vi "GetParameters.vi"() -> ()   [LabVIEW 2019]
panel:
  in  "Particle Measurements () ( Analysis 1) 2":dbl[][](array[numeric])=[[-56.76927788622368, -45.1835918273996, 105.49419358199933], [-30.750625061451895, -44.325520815009625, 68.38552020511543], [-2.1334363725101984, -41.244912471531386, 76.37528039980916], [29.421996518985512, -37.122571270909646, 66.76480625926112], [60.274191851517, -32.079988846679804, 77.89870639104257], [-27.384001212853015, -15.978175056162065, 86.41531854069336], [-57.12939186077779, -13.03821655068185, 95.19110987959867], [0.8157806454249426, -11.537585106806365, 62.65946754704529], [64.98159237148258, -10.313960473940636, 69.99468128482164], [32.817069309857175, -8.540823667699138, 60.761895469821624], [-27.702412887676708, 9.579157204985355, 75.19141634191074], [37.70198789537908, 10.266392184363795, 79.57588918149607], [4.765820750936916, 14.081942717017705, 68.51007357972752], [70.76309958374665, 15.0790537252041, 75.75366895030213], [-57.414383042714164, 15.41503234985349, 118.75231783795783], [38.63309694823678, 26.53758397944904, 71.30269833859165], [6.772199998928159, 31.011934793632058, 85.69802266359905], [73.41514437007658, 32.69142082569389, 70.93244311358723], [-24.768202720713113, 34.61278172695657, 103.9423369146022], [-57.24809342732071, 38.73521730856287, 115.82572787967626], [44.20007179514008, 45.43219064427871, 19.51567546366857], [79.96818037855478, 49.88188093239065, 32.063710672745785], [8.120161023706626, 52.661005797649594, 173.15722658736857], [-57.72569267153209, 55.966495303633685, 93.82758352841635], [-23.250568280228087, 59.94125217156932, 90.95001222194976]] format="%.2f"
  out "appended array 3":cluster{dbl, dbl}[][](array[cluster])
  out "MatrixPoint":cluster{dbl, dbl}[][](array[cluster])
  out "appended array":cluster{"X":dbl, "Y":dbl}[][](array[cluster])
  out "Number of Particles":i32
  out "CalImgOut":T1(plugin-control)
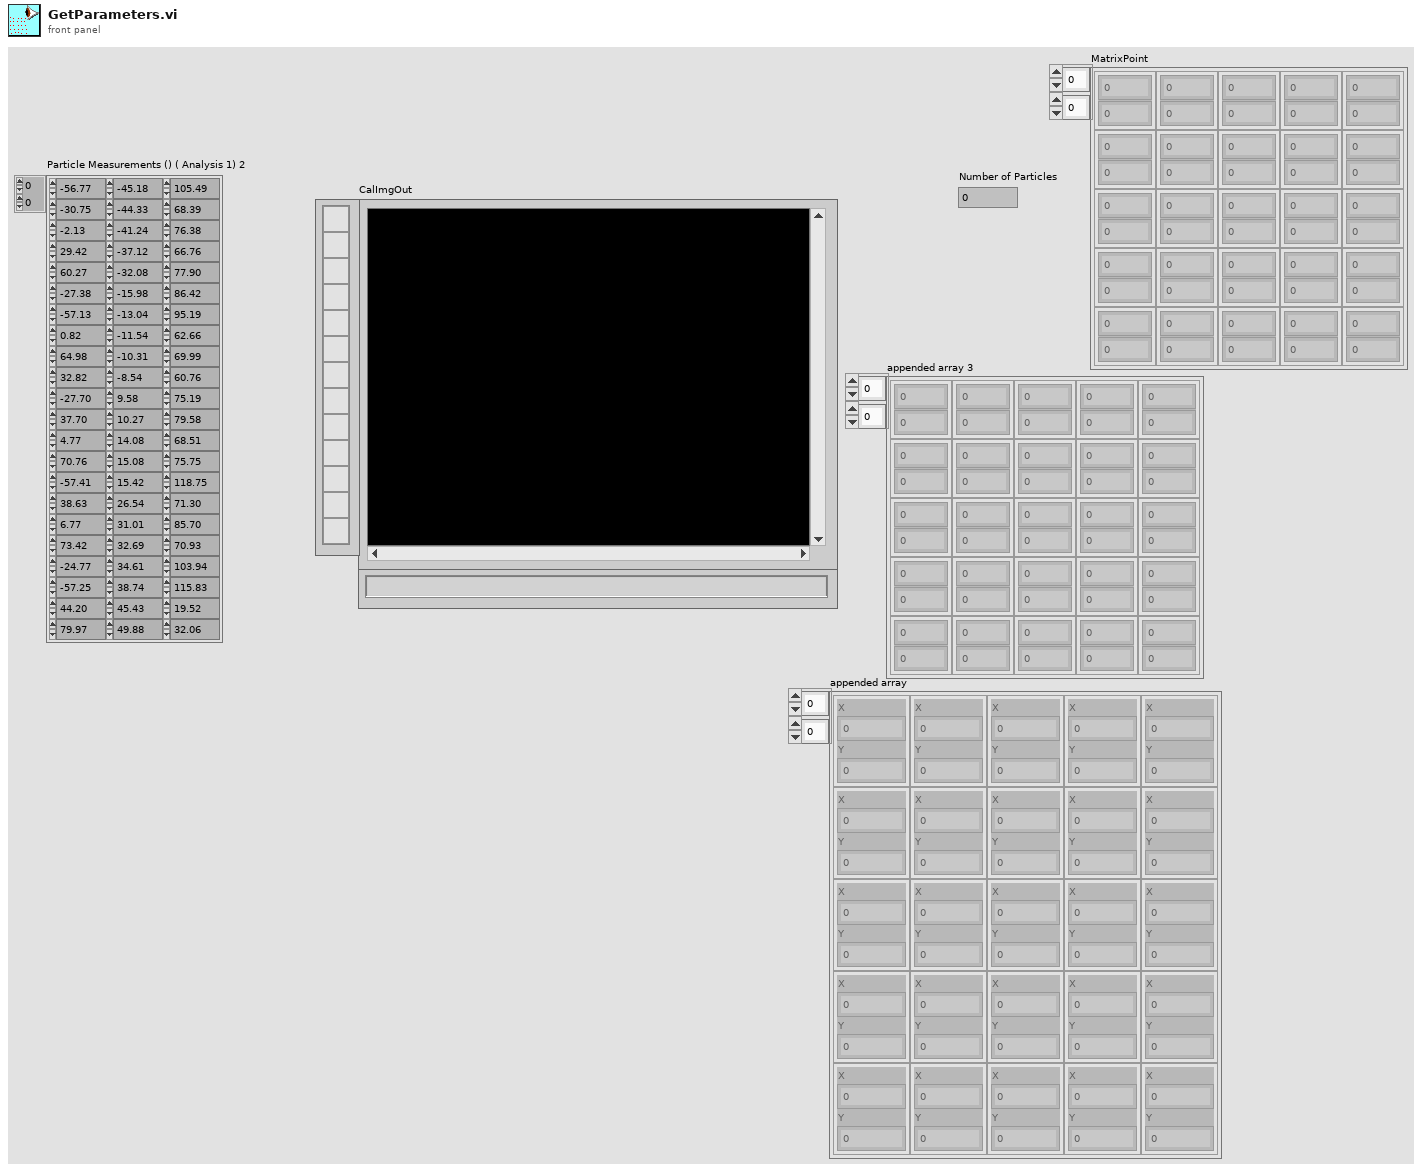
[diagram p1: front panel]
types:
  T1 = typedef "IMAQ Image.ctl" = refnum<image>
  T2 = typedef "Image Type" = u32
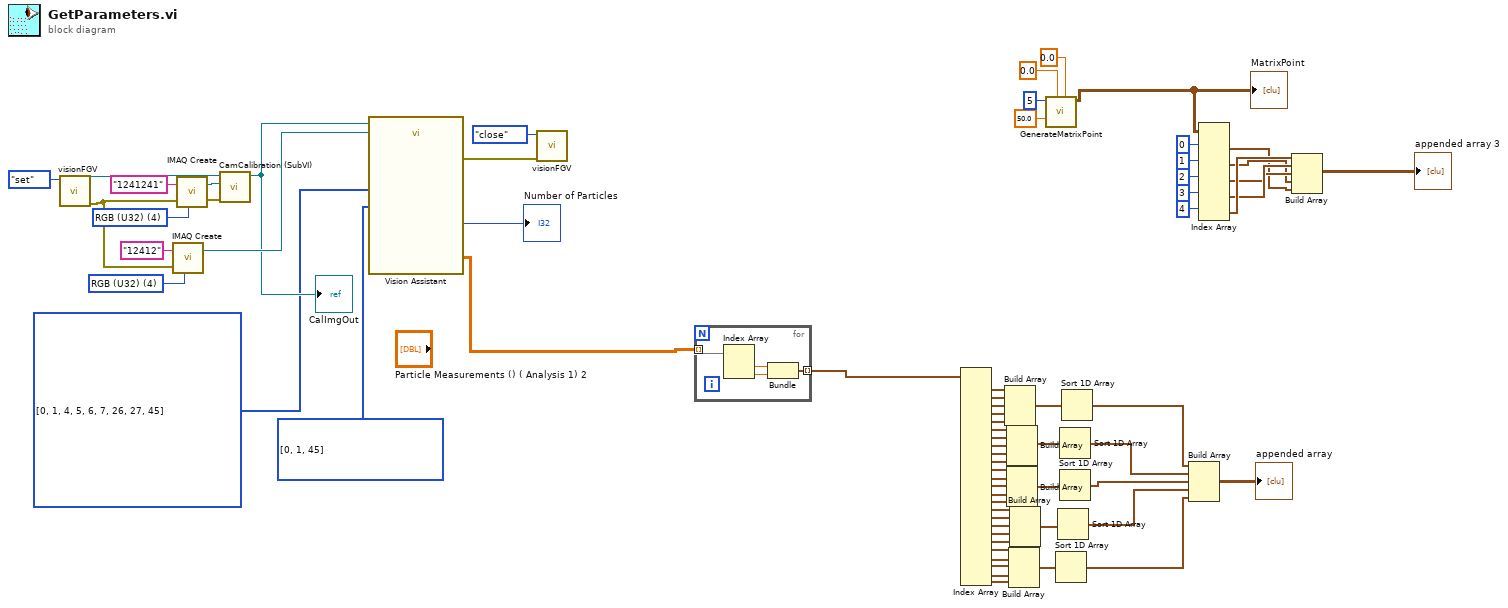
[diagram p0: block diagram]
diagram:
  w55 = i32[] [0, 1, 45] items=["Center of Mass X", "Center of Mass Y", "First Pixel X", "First Pixel Y", "Bounding Rect Left", "Bounding Rect Top", "Bounding Rect Right", "Bounding Rect Bottom", "Max Feret Diameter Start X", "Max Feret Diameter Start Y", "Max Feret Diameter End X", "Max Feret Diameter End Y", "Max Horiz. Segment Length Left", "Max Horiz. Segment Length Right", "Max Horiz. Segment Length Row", "-", "Bounding Rect Width", "Bounding Rect Height", "Bounding Rect Diagonal", "Perimeter", "Convex Hull Perimeter", "Holes' Perimeter", "Max Feret Diameter", "Equivalent Ellipse Major Axis", "Equivalent Ellipse Minor Axis", "Equivalent Ellipse Minor Axis (Feret)", "Equivalent Rect Long Side", "Equivalent Rect Short Side", "Equivalent Rect Diagonal", "Equivalent Rect Short Side (Feret)", "Average Horiz. Segment Length", "Average Vert. Segment Length", "Hydraulic Radius", "Waddel Disk Diameter", "-", "Area", "Holes' Area", "Particle & Holes' Area", "Convex Hull Area", "Image Area", "-", "Number of Holes", "Number of Horiz. Segments", "Number of Vert. Segments", "-", "Orientation", "Max Feret Diameter Orientation", "-", "% Area/Image Area", "% Area/(Particle & Holes' Area)", "Ratio of Equivalent Ellipse Axes", "Ratio of Equivalent Rect Sides", "-", "Elongation Factor", "Compactness Factor", "Heywood Circularity Factor", "Type Factor", "-", "Sum X", "Sum Y", "Sum XX", "Sum XY", "Sum YY", "Sum XXX", "Sum XXY", "Sum XYY", "Sum YYY", "-", "Moment of Inertia XX", "Moment of Inertia XY", "Moment of Inertia YY", "Moment of Inertia XXX", "Moment of Inertia XXY", "Moment of Inertia XYY", "Moment of Inertia YYY", "Norm. Moment of Inertia XX", "Norm. Moment of Inertia XY", "Norm. Moment of Inertia YY", "Norm. Moment of Inertia XXX", "Norm. Moment of Inertia XXY", "Norm. Moment of Inertia XYY", "Norm. Moment of Inertia YYY", "Hu Moment 1", "Hu Moment 2", "Hu Moment 3", "Hu Moment 4", "Hu Moment 5", "Hu Moment 6", "Hu Moment 7"] ("Real-World Measurements (Particle Analysis 1)")
  w56 = i32[] [0, 1, 4, 5, 6, 7, 26, 27, 45] items=["Center of Mass X", "Center of Mass Y", "First Pixel X", "First Pixel Y", "Bounding Rect Left", "Bounding Rect Top", "Bounding Rect Right", "Bounding Rect Bottom", "Max Feret Diameter Start X", "Max Feret Diameter Start Y", "Max Feret Diameter End X", "Max Feret Diameter End Y", "Max Horiz. Segment Length Left", "Max Horiz. Segment Length Right", "Max Horiz. Segment Length Row", "-", "Bounding Rect Width", "Bounding Rect Height", "Bounding Rect Diagonal", "Perimeter", "Convex Hull Perimeter", "Holes' Perimeter", "Max Feret Diameter", "Equivalent Ellipse Major Axis", "Equivalent Ellipse Minor Axis", "Equivalent Ellipse Minor Axis (Feret)", "Equivalent Rect Long Side", "Equivalent Rect Short Side", "Equivalent Rect Diagonal", "Equivalent Rect Short Side (Feret)", "Average Horiz. Segment Length", "Average Vert. Segment Length", "Hydraulic Radius", "Waddel Disk Diameter", "-", "Area", "Holes' Area", "Particle & Holes' Area", "Convex Hull Area", "Image Area", "-", "Number of Holes", "Number of Horiz. Segments", "Number of Vert. Segments", "-", "Orientation", "Max Feret Diameter Orientation", "-", "% Area/Image Area", "% Area/(Particle & Holes' Area)", "Ratio of Equivalent Ellipse Axes", "Ratio of Equivalent Rect Sides", "-", "Elongation Factor", "Compactness Factor", "Heywood Circularity Factor", "Type Factor", "-", "Sum X", "Sum Y", "Sum XX", "Sum XY", "Sum YY", "Sum XXX", "Sum XXY", "Sum XYY", "Sum YYY", "-", "Moment of Inertia XX", "Moment of Inertia XY", "Moment of Inertia YY", "Moment of Inertia XXX", "Moment of Inertia XXY", "Moment of Inertia XYY", "Moment of Inertia YYY", "Norm. Moment of Inertia XX", "Norm. Moment of Inertia XY", "Norm. Moment of Inertia YY", "Norm. Moment of Inertia XXX", "Norm. Moment of Inertia XXY", "Norm. Moment of Inertia XYY", "Norm. Moment of Inertia YYY", "Hu Moment 1", "Hu Moment 2", "Hu Moment 3", "Hu Moment 4", "Hu Moment 5", "Hu Moment 6", "Hu Moment 7"] ("Pixel Measurements (Particle Analysis 1)")
  w68 = T2 4 items=["Grayscale (U8)", "Grayscale (I16)", "Grayscale (SGL)", "Complex (CSG)", "RGB (U32)", "HSL (U32)", "RGB (U64)", "Grayscale (U16)"] ("Image Type")
  w69 = T2 4 items=["Grayscale (U8)", "Grayscale (I16)", "Grayscale (SGL)", "Complex (CSG)", "RGB (U32)", "HSL (U32)", "RGB (U64)", "Grayscale (U16)"] ("Image Type")
  n1 = call "visionFGV.vi"("Function"=enum16{"set", "read", "close"}."set") -> ("error out"=w63:errorcluster, "Image Out fgv"=w61:T1)  [unwired: 9 in]
  n2 = call "IMAQ Create"("Image Name"="12412", "Image Type"=w68, "error in (no error)"=w63) -> ("New Image"=w66:T1)  [unwired: 2 in, 1 out]
  n3 = call "IMAQ Create"("Image Name"="1241241", "Image Type"=w69, "error in (no error)"=w63) -> ("New Image"=w65:T1, "error out"=w62:errorcluster)  [unwired: 2 in]
  n4 = call "CamCalibration (SubVI).vi"("error in"=w62, "Image Dst"=w65, "Image In"=w61) -> ("Image Out"=w60:T1)  [unwired: 7 in, 1 out]
  "CalImgOut" <- w60
  n5 = call "Vision Assistant"("Image In"=w60, "Image Dst"=w66, "Pixel Measurements (Particle Analysis 1)"=w56, "Real-World Measurements (Particle Analysis 1)"=w55) -> ("Particle Measurements (Real-World) (Particle Analysis 1)"=w1:dbl[][], "Number of Particles (Particle Analysis 1)"=→"Number of Particles":i32, "error out"=w59:errorcluster)  [unwired: 19 in, 2 out]
  n6 = call "visionFGV.vi"("Error In"=w59, "Function"=enum16{"set", "read", "close"}."close") -> ()  [unwired: 8 in, 2 out]
  n7 = for {
    tunnel: w1 -> [w74] mode=indexing
    tunnel: [w71] -> w27 mode=indexing
    n8 = Index Array(array=w74) -> (element #1=w73:dbl, element #2=w72:dbl)  [unwired: 2 in]
    n9 = Bundle("Numeric"=w73, "Numeric"=w72) -> (w71:cluster{"Numeric":dbl, "Numeric":dbl})  [unwired: 1 in]
  }
  n10 = Index Array(array=w27) -> (element #1=w28:cluster{"Numeric":dbl, "Numeric":dbl}, element #2=w38:cluster{"Numeric":dbl, "Numeric":dbl}, element #3=w37:cluster{"Numeric":dbl, "Numeric":dbl}, element #4=w36:cluster{"Numeric":dbl, "Numeric":dbl}, element #5=w35:cluster{"Numeric":dbl, "Numeric":dbl}, element #6=w34:cluster{"Numeric":dbl, "Numeric":dbl}, element #7=w33:cluster{"Numeric":dbl, "Numeric":dbl}, element #8=w30:cluster{"Numeric":dbl, "Numeric":dbl}, element #9=w32:cluster{"Numeric":dbl, "Numeric":dbl}, element #10=w31:cluster{"Numeric":dbl, "Numeric":dbl}, element #11=w24:cluster{"Numeric":dbl, "Numeric":dbl}, element #12=w23:cluster{"Numeric":dbl, "Numeric":dbl}, element #13=w22:cluster{"Numeric":dbl, "Numeric":dbl}, element #14=w21:cluster{"Numeric":dbl, "Numeric":dbl}, element #15=w20:cluster{"Numeric":dbl, "Numeric":dbl}, element #16=w19:cluster{"Numeric":dbl, "Numeric":dbl}, element #17=w18:cluster{"Numeric":dbl, "Numeric":dbl}, element #18=w17:cluster{"Numeric":dbl, "Numeric":dbl}, element #19=w16:cluster{"Numeric":dbl, "Numeric":dbl}, element #20=w15:cluster{"Numeric":dbl, "Numeric":dbl}, element #21=w14:cluster{"Numeric":dbl, "Numeric":dbl}, element #22=w13:cluster{"Numeric":dbl, "Numeric":dbl}, element #23=w12:cluster{"Numeric":dbl, "Numeric":dbl}, element #24=w11:cluster{"Numeric":dbl, "Numeric":dbl}, element #25=w10:cluster{"Numeric":dbl, "Numeric":dbl})  [unwired: 25 in]
  n11 = Build Array(w28, w38, w37, w36, w35) -> (w26:cluster{"Numeric":dbl, "Numeric":dbl}[])
  n12 = Build Array(w34, w33, w30, w32, w31) -> (w25:cluster{"Numeric":dbl, "Numeric":dbl}[])
  n13 = Build Array(w24, w23, w22, w21, w20) -> (w7:cluster{"Numeric":dbl, "Numeric":dbl}[])
  n14 = Build Array(w14, w13, w12, w11, w10) -> (w9:cluster{"Numeric":dbl, "Numeric":dbl}[])
  n15 = Build Array(w19, w18, w17, w16, w15) -> (w8:cluster{"Numeric":dbl, "Numeric":dbl}[])
  n16 = call "GenerateMatrixPoint.vi"("YOffSet"=0.0, "XOffSet"=0.0, "Pitch"=50.0, "MatrixSize"=5) -> ("MatrixPoint"=w39:cluster{dbl, dbl}[][])  [unwired: 6 in, 1 out]
  "MatrixPoint" <- w39
  n17 = Sort 1D Array(array=w9) -> (sorted array=w2:cluster{"Numeric":dbl, "Numeric":dbl}[])
  n18 = Sort 1D Array(array=w8) -> (sorted array=w3:cluster{"Numeric":dbl, "Numeric":dbl}[])
  n19 = Sort 1D Array(array=w25) -> (sorted array=w5:cluster{"Numeric":dbl, "Numeric":dbl}[])
  n20 = Sort 1D Array(array=w7) -> (sorted array=w4:cluster{"Numeric":dbl, "Numeric":dbl}[])
  n21 = Sort 1D Array(array=w26) -> (sorted array=w6:cluster{"Numeric":dbl, "Numeric":dbl}[])
  n22 = Build Array(w6, w5, w4, w3, w2) -> (→"appended array":cluster{"Numeric":dbl, "Numeric":dbl}[][])
  n23 = Index Array(array=w39, index (row) #1=0 ("index (row)"), index (row) #2=1 ("index (row)"), index (row) #3=2 ("index (row)"), index (row) #4=3 ("index (row)"), index (row) #5=4 ("index (row)")) -> (element #1=w41:cluster{dbl, dbl}[], element #2=w42:cluster{dbl, dbl}[], element #3=w43:cluster{dbl, dbl}[], element #4=w44:cluster{dbl, dbl}[], element #5=w45:cluster{dbl, dbl}[])  [unwired: 5 in]
  n24 = Build Array(w45, w44, w43, w42, w41) -> (→"appended array 3":cluster{dbl, dbl}[][])
